vi "PDLM_DllPath_global.vi"() -> ()   [LabVIEW 2019]
panel:
  in  "DllPath":path=path "P:/hagen/PDLM/API/Win64/Release/pdlm_lib.dll"
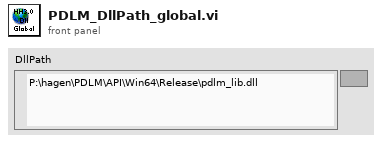
[diagram p1: front panel]
diagram:
